vi "Monty-Hall.vi"() -> ()   [LabVIEW 2021]
uses:
  <vilib>/Platform/TimedLoop/XDataNode/timing_clust.ctl
  <vilib>/Platform/TimedLoop/XDataNode/nitl_modes.ctl
  <vilib>/Platform/TimedLoop/XDataNode/wakeup.ctl
  <vilib>/platform/TimedLoop/XDataNode/XDataNode.xnode
  <vilib>/Platform/TimedLoop/XDataNode/XDNodeRunTimeDep.lvlib
panel:
  out "Manual Wins":cluster{i32[], i32[]}[](graph)
  out "Manual Win":bool
  in  "Stay":bool
  in  "Switch":bool
  in  "?":bool
  in  "?":bool
  in  "?":bool
  in  "?":bool
  in  "?":bool
  in  "?":bool
  in  "?":bool
  in  "?":bool
  in  "?":bool
  in  "?":bool
  in  "Mode":i8(slide) min=0 max=2 step=1 scale=0.0..2.0
  out "Simulated Win":bool
  out "Simulated Odds":cluster{i32[], dbl[]}[](graph)
  in  "Door Count":dbl=3.0 min=3.0 max=10.0 step=1.0
  in  "Trial Count":dbl=1.0 min=1.0 step=1.0
  # "(note: set slider before starting VI)"
  # "In play mode, click a door, then either click switch or stay to remain with your original choice or swap to the other remaining door (Monty Hall Problem)"
  # "(note: VI automatically loops in play mode)"
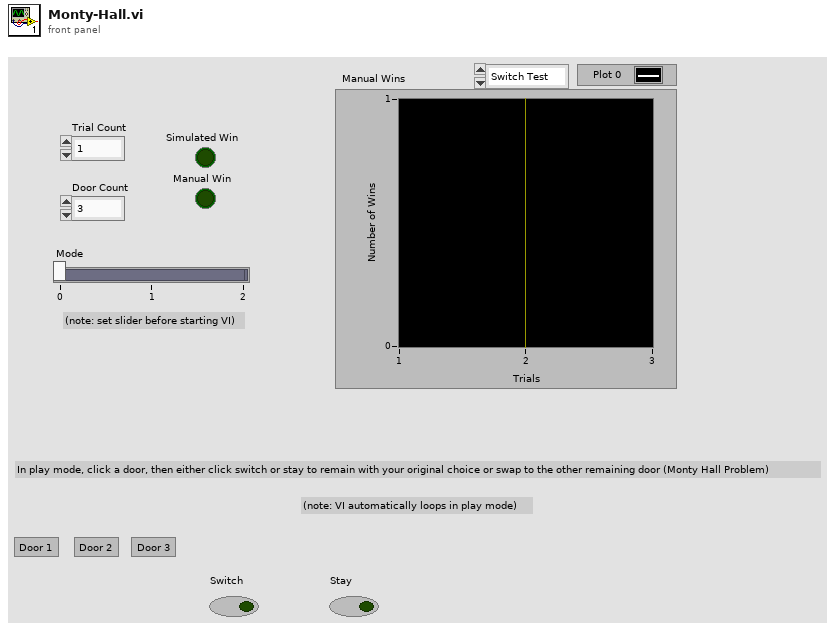
[diagram p1: front panel]
types:
  T1 = typedef "XDNodeRunTimeDep.lvlib/timing_clust.ctl" = cluster{"Expected End [f-1]":u64, "Actual End [f-1]":u64, "Finished Late? [f-1]":bool, "Expected End [i-1]":u64, "Actual End [i-1]":u64, "Finished Late? [i-1]":bool, "Expected Start [i]":u64, "Actual Start [i]":u64, "Expected Start [f]":u64, "Actual Start [f]":u64, "Source Name":string, "Structure Name":string, "Period":i64, "Deadline":i64, "Offset":i64, "Start":i64, "Priority":i32, "Timeout":i32, "Mode":T2, "Wakeup Reason":T3, "Error":errorcluster, "Source Type":string, "Secondary Source Type":string, "Global End Time":u64, "Global Start Time":u64, "Frame Duration":u64, "Iteration Duration":u64, "Assigned CPU":i32, "I/O Scan Engine Mode":u32}
  T2 = typedef "XDNodeRunTimeDep.lvlib/nitl_modes.ctl" = enum32{"No Change", "Process missed periods, maintain original phase", "Discard missed periods, maintain original phase", "Process missed periods, ignore original phase", "Discard missed periods, ignore original phase"}
  T3 = typedef "XDNodeRunTimeDep.lvlib/wakeup.ctl" = enum32{"Normal", "Aborted", "Asynchronous wakeup", "Timing source error", "Timed loop error", "Timeout"}
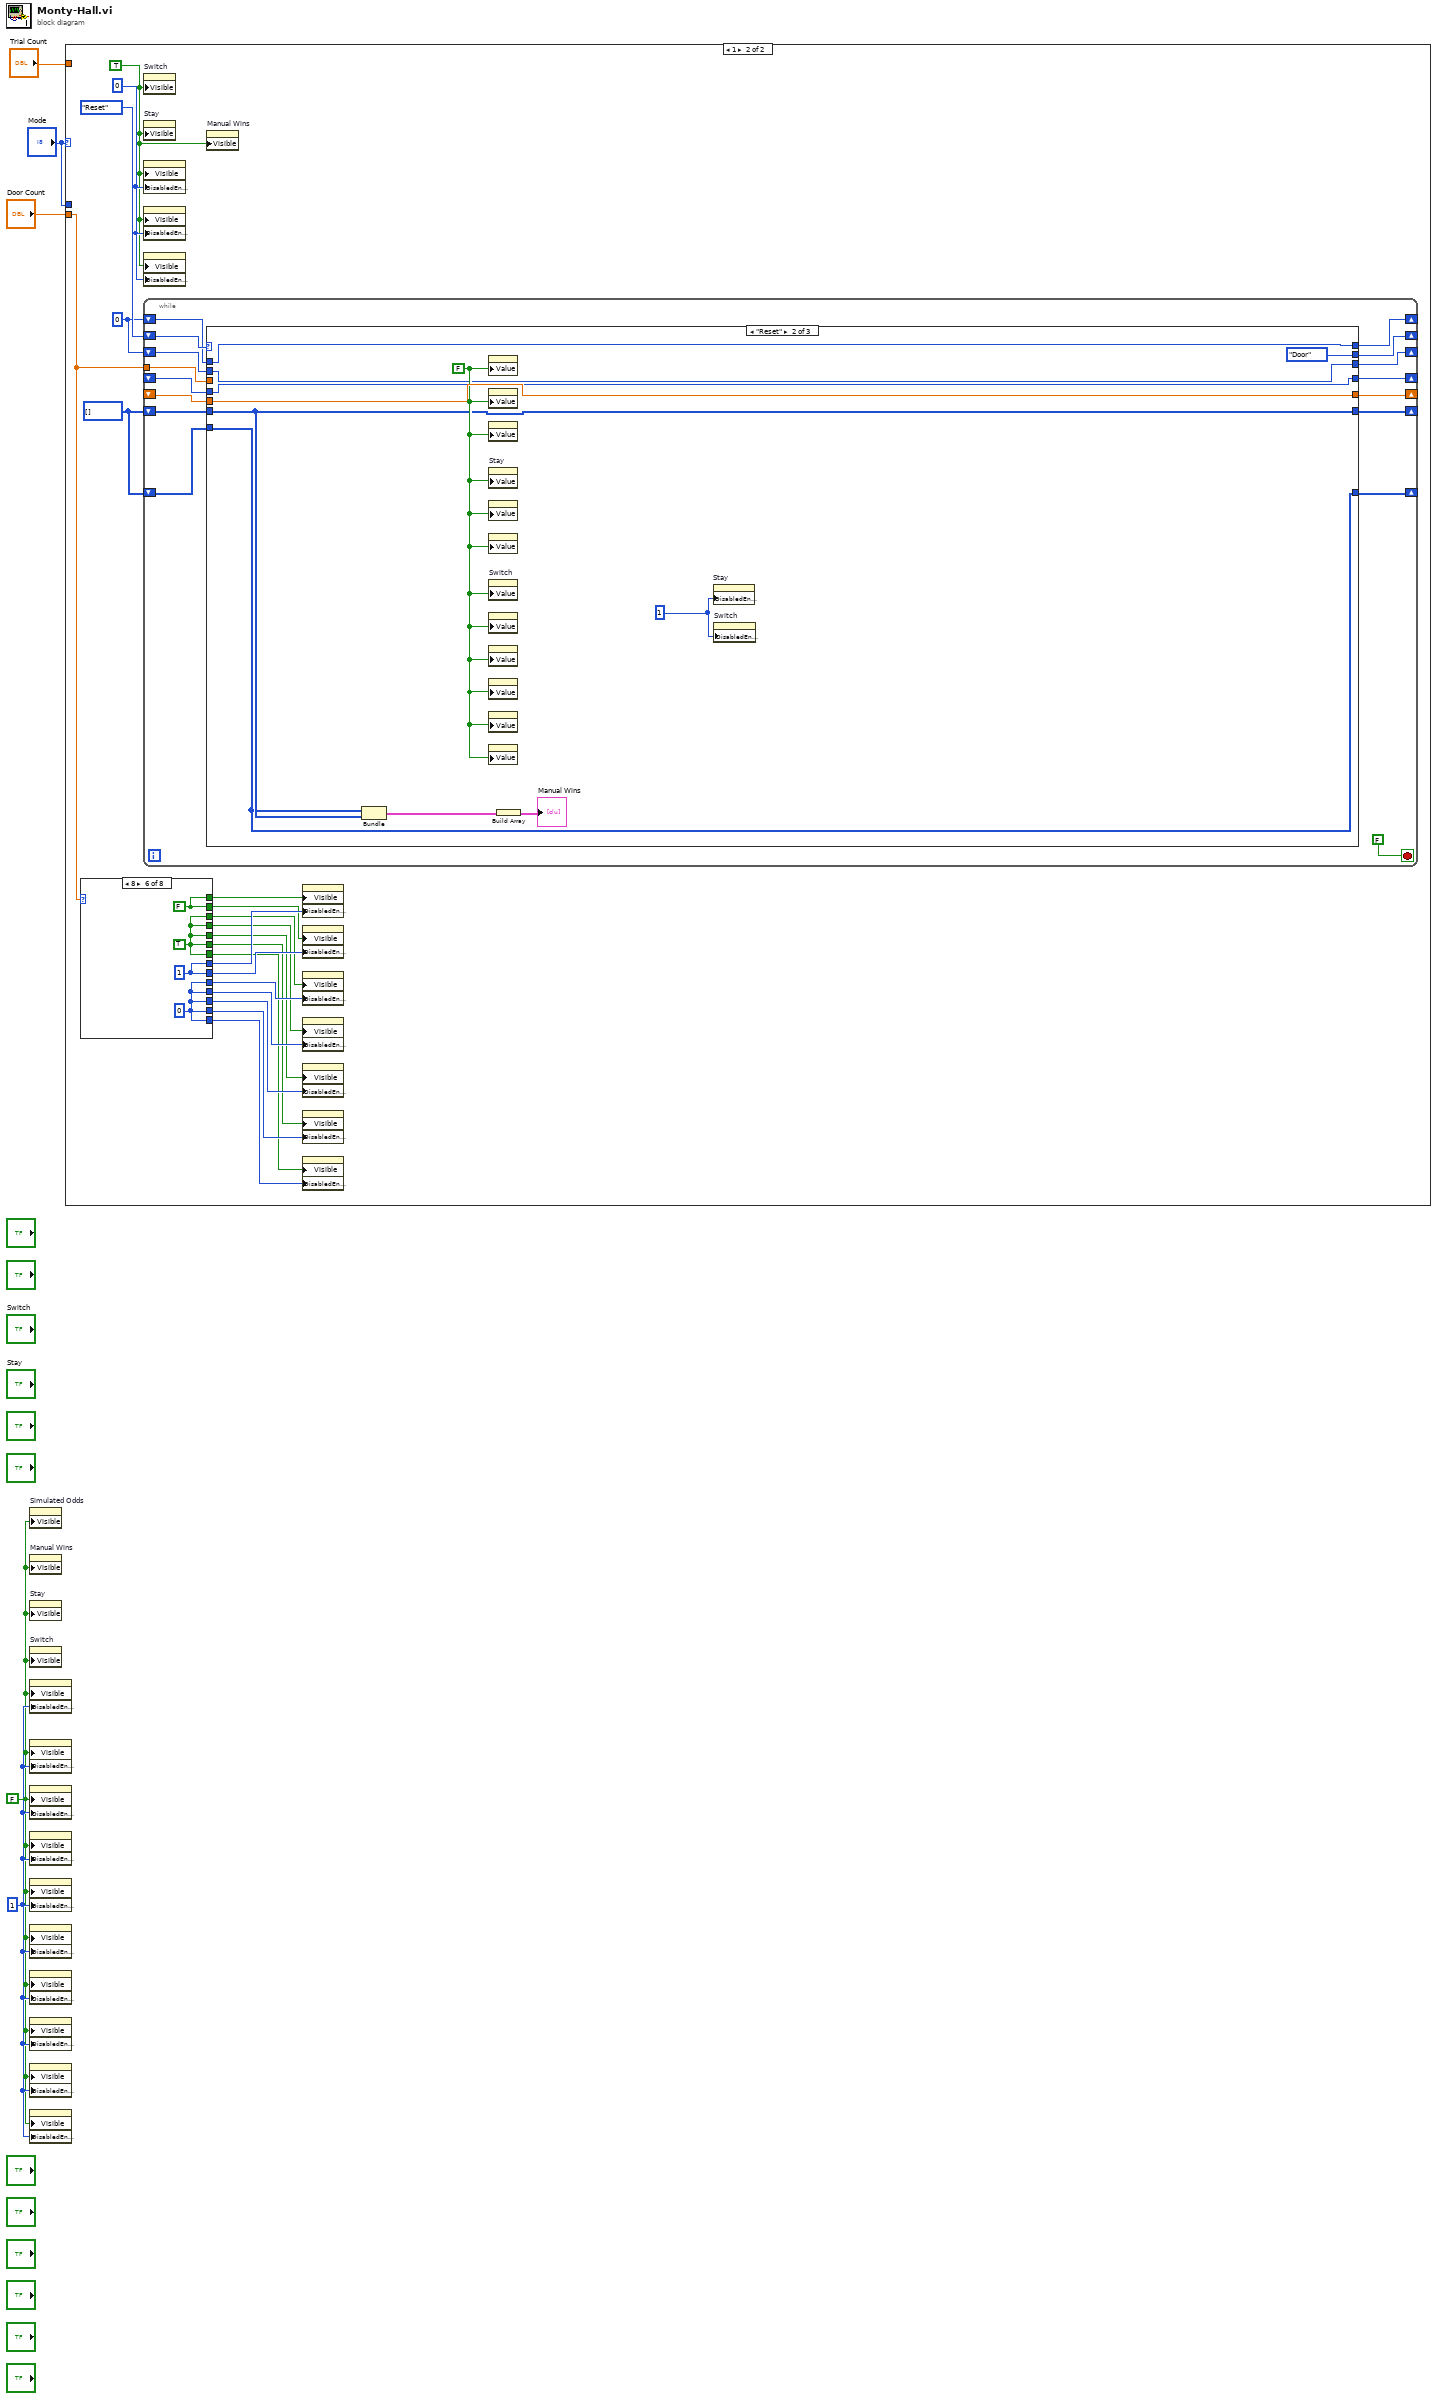
[diagram p0: block diagram]
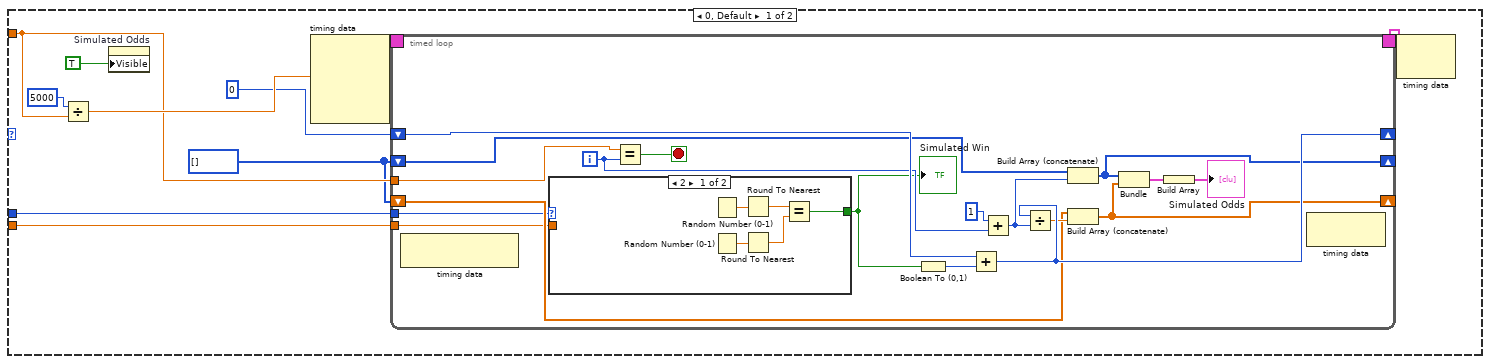
[diagram p2: hidden frame]
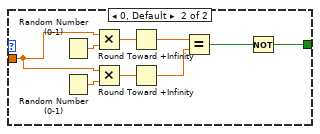
[diagram p3: hidden frame]
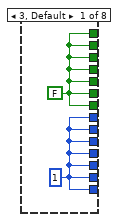
[diagram p4: hidden frame]
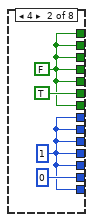
[diagram p5: hidden frame]
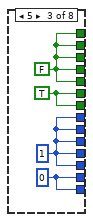
[diagram p6: hidden frame]
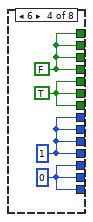
[diagram p7: hidden frame]
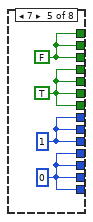
[diagram p8: hidden frame]
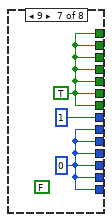
[diagram p9: hidden frame]
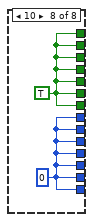
[diagram p10: hidden frame]
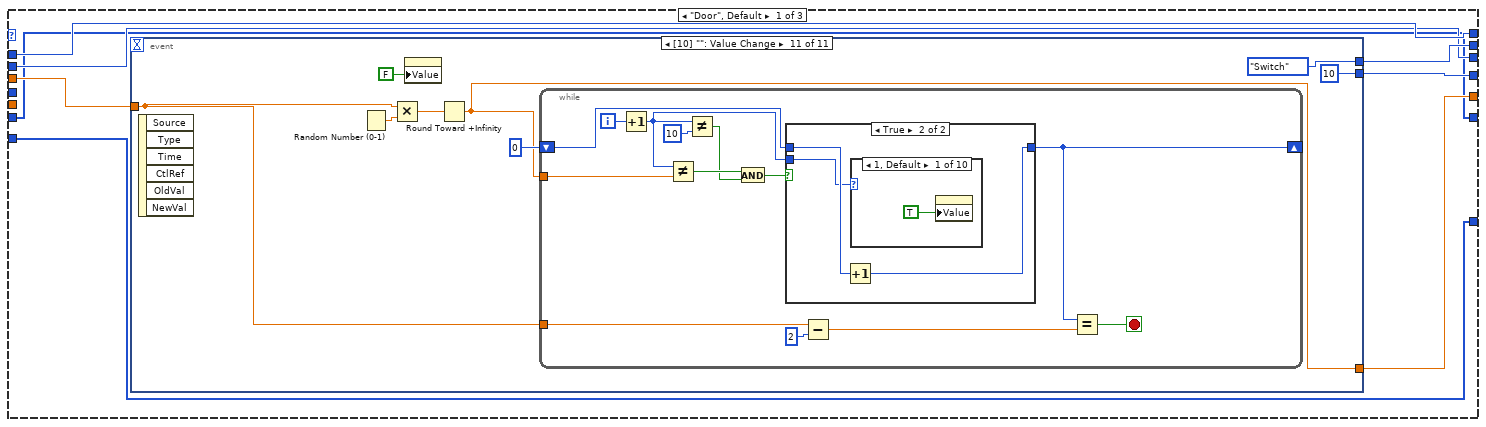
[diagram p11: hidden frame]
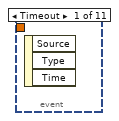
[diagram p12: hidden frame]
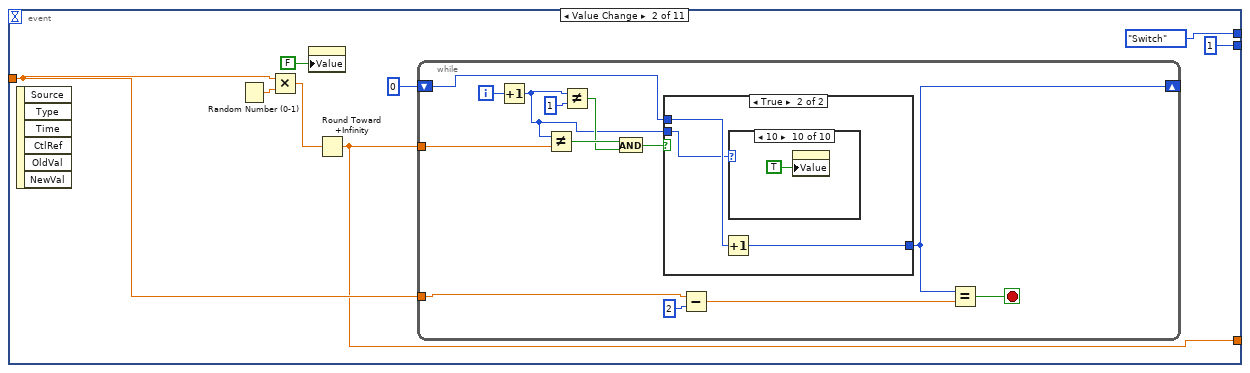
[diagram p13: hidden frame]
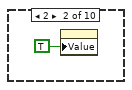
[diagram p16: hidden frame]
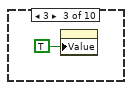
[diagram p17: hidden frame]
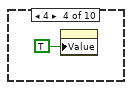
[diagram p18: hidden frame]
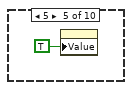
[diagram p19: hidden frame]
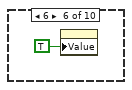
[diagram p20: hidden frame]
diagram:
  w3 = 1
  w1 = FALSE
  n1 = property on="Simulated Odds" class="XYGraph (strict)"("Visible"=w1) -> ()  [unwired: 2 in, 2 out]
  n2 = property on="Manual Wins" class="XYGraph (strict)"("Visible"=w1) -> ()  [unwired: 2 in, 2 out]
  n3 = property on="Stay" class="Bool (strict)"("Visible"=w1) -> ()  [unwired: 2 in, 2 out]
  n4 = property on="Switch" class="Bool (strict)"("Visible"=w1) -> ()  [unwired: 2 in, 2 out]
  n5 = property class="Bool (strict)"("Visible"=w1, "DisabledEnum"=w3) -> ()  [unwired: 2 in, 2 out]
  n6 = property class="Bool (strict)"("Visible"=w1, "DisabledEnum"=w3) -> ()  [unwired: 2 in, 2 out]
  n7 = property class="Bool (strict)"("Visible"=w1, "DisabledEnum"=w3) -> ()  [unwired: 2 in, 2 out]
  n8 = property class="Bool (strict)"("Visible"=w1, "DisabledEnum"=w3) -> ()  [unwired: 2 in, 2 out]
  n9 = property class="Bool (strict)"("Visible"=w1, "DisabledEnum"=w3) -> ()  [unwired: 2 in, 2 out]
  n10 = property class="Bool (strict)"("Visible"=w1, "DisabledEnum"=w3) -> ()  [unwired: 2 in, 2 out]
  n11 = property class="Bool (strict)"("Visible"=w1, "DisabledEnum"=w3) -> ()  [unwired: 2 in, 2 out]
  n12 = property class="Bool (strict)"("Visible"=w1, "DisabledEnum"=w3) -> ()  [unwired: 2 in, 2 out]
  n13 = property class="Bool (strict)"("Visible"=w1, "DisabledEnum"=w3) -> ()  [unwired: 2 in, 2 out]
  n14 = property class="Bool (strict)"("Visible"=w1, "DisabledEnum"=w3) -> ()  [unwired: 2 in, 2 out]
  n15 = case shown="1" "Mode" {
    tunnel: "Trial Count" -> [w11 _]
    tunnel: "Door Count" -> [w10 w72]
    tunnel: "Mode" -> [w7 _]
    frame 0, Default {
      w8 = i32[] []
      n16 = Divide(x=5000, y=w11) -> (x/y=w12:dbl)
      n17 = property on="Simulated Odds" class="XYGraph (strict)"("Visible"=TRUE) -> ()  [unwired: 2 in, 2 out]
      n18 = node-c288(w12) -> (w14:T1)  [unwired: 3 in]
      n19 = timed-loop {
        timing: w14 -> [_]
        timing-out: [_] -> w13
        shift-right: [w23] -> _
        shift-left: w8 -> [w22]
        tunnel: w11 -> [w33]
        tunnel: w10 -> [w18]
        shift-right: [w29] -> _
        shift-left: 0 -> [w30]
        shift-right: [w20] -> _
        shift-left: w8 -> [w19]
        tunnel: w7 -> [w16]
        i -> [w27]
        stop <- w32 stop-if-true
        n20 = node-c288() -> ()  [unwired: 1 in, 1 out]
        n21 = case shown="2" w16 {
          tunnel: w18 -> [_ w43]
          tunnel: [w34 w39] -> w17
          frame 2 {
            n22 = Random Number (0-1)() -> (number: 0 to 1=w38:dbl)
            n23 = Random Number (0-1)() -> (number: 0 to 1=w37:dbl)
            n24 = Round To Nearest(number=w38) -> (nearest integer value=w36:dbl)
            n25 = Round To Nearest(number=w37) -> (nearest integer value=w35:dbl)
            n26 = Equal?(x=w36, y=w35) -> (x = y?=w34:bool)
          }
          frame 0, Default {
            n27 = Random Number (0-1)() -> (number: 0 to 1=w47:dbl)
            n28 = Random Number (0-1)() -> (number: 0 to 1=w45:dbl)
            n29 = Multiply(x=w43, y=w47) -> (x*y=w46:dbl)
            n30 = Multiply(x=w43, y=w45) -> (x*y=w44:dbl)
            n31 = Round Toward +Infinity(x=w46) -> (ceil(x): smallest int >= x=w42:dbl)
            n32 = Round Toward +Infinity(x=w44) -> (ceil(x): smallest int >= x=w41:dbl)
            n33 = Equal?(x=w42, y=w41) -> (x = y?=w40:bool)
            n34 = Not(x=w40) -> (.not. x?=w39:bool)
          }
        }
        "Simulated Win" <- w17
        n35 = Equal?(x=w33, y=w27) -> (x = y?=w32:bool)
        n36 = Boolean To (0,1)(Boolean=w17) -> (0, 1=w31:i16)
        n37 = Add(x=w30, y=w31) -> (x+y=w29:i32)
        n38 = Add(x=1, y=w27) -> (x+y=w21:i32)
        n39 = Divide(x=w29, y=w21) -> (x/y=w24:dbl)
        n40 = Build Array (concatenate)(w19, w21) -> (w20:i32[])
        n41 = Build Array (concatenate)(w22, w24) -> (w23:dbl[])
        n42 = Bundle(w20, w23) -> (w26:cluster{i32[], dbl[]})  [unwired: 1 in]
        n43 = Build Array(w26) -> (→"Simulated Odds":cluster{i32[], dbl[]}[])
        n44 = node-c288() -> ()  [unwired: 1 in, 1 out]
      }
      n45 = node-c288(w13) -> ()  [unwired: 1 out]
    }
    frame 1 {
      w55 = i32[] []
      w56 = 0
      w54 = TRUE
      w73 = 0
      n46 = case shown="8" w72 {
        tunnel: [w75 0 w82 w87 w88 w92 w98 w99] -> w71
        tunnel: [w75 w77 w82 w87 w88 w92 w98 w99] -> w70
        tunnel: [w75 w77 w81 w87 w88 w92 w98 w99] -> w69
        tunnel: [w75 w77 w81 w85 w88 w92 w98 w99] -> w68
        tunnel: [w75 w77 w81 w85 w89 w92 w98 w99] -> w67
        tunnel: [w75 w77 w81 w85 w89 w94 w98 w99] -> w66
        tunnel: [w75 w77 w81 w85 w89 w94 1 w99] -> w65
        tunnel: [w74 TRUE w83 w86 w91 w95 w96 w100] -> w64
        tunnel: [w74 w76 w83 w86 w91 w95 w96 w100] -> w63
        tunnel: [w74 w76 w80 w86 w91 w95 w96 w100] -> w62
        tunnel: [w74 w76 w80 w84 w91 w95 w96 w100] -> w61
        tunnel: [w74 w76 w80 w84 w90 w95 w96 w100] -> w60
        tunnel: [w74 w76 w80 w84 w90 w93 w96 w100] -> w59
        tunnel: [w74 w76 w80 w84 w90 w93 w96 w100] -> w58
        frame 3, Default {
          w74 = FALSE
          w75 = 1
        }
        frame 4 {
          w76 = FALSE
          w77 = 1
        }
        frame 5 {
          w80 = FALSE
          w81 = 1
          w83 = TRUE
          w82 = 0
        }
        frame 6 {
          w84 = FALSE
          w85 = 1
          w86 = TRUE
          w87 = 0
        }
        frame 7 {
          w90 = FALSE
          w89 = 1
          w91 = TRUE
          w88 = 0
        }
        frame 8 {
          w93 = FALSE
          w94 = 1
          w95 = TRUE
          w92 = 0
        }
        frame 9 {
          (unwired) FALSE
          w96 = TRUE
          w98 = 0
        }
        frame 10 {
          w100 = TRUE
          w99 = 0
        }
      }
      n47 = property on="Switch" class="Bool (strict)"("Visible"=w54) -> ()  [unwired: 2 in, 2 out]
      n48 = property on="Stay" class="Bool (strict)"("Visible"=w54) -> ()  [unwired: 2 in, 2 out]
      n49 = property class="Bool (strict)"("Visible"=w54, "DisabledEnum"=w73) -> ()  [unwired: 2 in, 2 out]
      n50 = property class="Bool (strict)"("Visible"=w54, "DisabledEnum"=w73) -> ()  [unwired: 2 in, 2 out]
      n51 = property class="Bool (strict)"("Visible"=w54, "DisabledEnum"=w73) -> ()  [unwired: 2 in, 2 out]
      n52 = while {
        tunnel: w72 -> [w115]
        shift-right: [w113] -> _
        shift-left: enum16{"Door", "Reset", "Switch"}."Reset" -> [w114]
        shift-right: [w112] -> _
        shift-left: _ -> [w111]
        shift-right: [w110] -> _
        shift-left: _ -> [w109]
        shift-right: [w105] -> _
        shift-left: w56 -> [w106]
        shift-right: [w107] -> _
        shift-left: w56 -> [w108]
        shift-right: [w101] -> _
        shift-left: w55 -> [w104]
        shift-right: [w102] -> _
        shift-left: w55 -> [w103]
        stop <- FALSE stop-if-true
        n53 = case shown="\"Reset\"" w114 {
          tunnel: w115 -> [w124 _ _]
          tunnel: [w123 enum16{"Door", "Reset", "Switch"}."Door" enum16{"Door", "Reset", "Switch"}."Reset"] -> w113
          tunnel: [w122 w483 w497] -> w112
          tunnel: w111 -> [_ w483 w499]
          tunnel: [w121 w482 w497] -> w110
          tunnel: w109 -> [_ w482 w498]
          tunnel: w108 -> [w119 w478 w494]
          tunnel: [w119 w478 w489] -> w107
          tunnel: w106 -> [w120 w479 w492]
          tunnel: [w120 w479 w490] -> w105
          tunnel: w104 -> [w118 w475 w491]
          tunnel: w103 -> [w117 w476 w488]
          tunnel: [w117 w476 w487] -> w102
          tunnel: [w118 w475 w486] -> w101
          frame "Door", Default {
            n54 = event shown="[10] \"\": Value Change" {
              selector: _ -> [_ _ _ _ _ _ _ _ _ _ _]
              dyn-events: _ -> [_ _ _ _ _ _ _ _ _ _ _]
              timeout: _ -> [_ _ _ _ _ _ _ _ _ _ _]
              tunnel: w124 -> [_ w128 w159 w197 w232 w266 w301 w334 w371 w406 w441]
              tunnel: [_ enum16{"Door", "Reset", "Switch"}."Switch" enum16{"Door", "Reset", "Switch"}."Switch" enum16{"Door", "Reset", "Switch"}."Switch" enum16{"Door", "Reset", "Switch"}."Switch" enum16{"Door", "Reset", "Switch"}."Switch" enum16{"Door", "Reset", "Switch"}."Switch" enum16{"Door", "Reset", "Switch"}."Switch" enum16{"Door", "Reset", "Switch"}."Switch" enum16{"Door", "Reset", "Switch"}."Switch" enum16{"Door", "Reset", "Switch"}."Switch"] -> w123
              tunnel: [_ w127 w162 w196 w231 w267 w302 w337 w372 w407 w442] -> w122
              tunnel: [_ 1 2 3 4 5 6 7 8 9 10] -> w121
              event Timeout {
                n55 = event-data() -> ()  [unwired: 1 in, 3 out]
              }
              event Value Change {
                n56 = event-data() -> ()  [unwired: 1 in, 6 out]
                n57 = Random Number (0-1)() -> (number: 0 to 1=w131:dbl)
                n58 = Multiply(x=w128, y=w131) -> (x*y=w132:dbl)
                n59 = property class="Bool (strict)"("Value"=FALSE) -> ()  [unwired: 2 in, 2 out]
                n60 = Round Toward +Infinity(x=w132) -> (ceil(x): smallest int >= x=w127:dbl)
                n61 = while {
                  tunnel: w128 -> [w137]
                  tunnel: w127 -> [w145]
                  shift-right: [w139] -> _
                  shift-left: 0 -> [w140]
                  i -> [w134]
                  stop <- w135 stop-if-true
                  n62 = Increment(x=w134) -> (x+1=w133:i32)
                  n63 = Not Equal?(x=w133, y=w145) -> (x != y?=w144:bool)
                  n64 = Not Equal?(x=w133, y=1) -> (x != y?=w142:bool)
                  n65 = And(x=w144, y=w142) -> (x .and. y?=w141:bool)
                  n66 = case shown="True" w141 {
                    tunnel: w140 -> [w146 w149]
                    tunnel: [w146 w148] -> w139
                    tunnel: w133 -> [_ w147]
                    frame False {
                    }
                    frame True {
                      n67 = Increment(x=w149) -> (x+1=w148:i32)
                      n68 = case shown="10" w147 {
                        frame 1, Default {
                        }
                        frame 2 {
                          n69 = property class="Bool (strict)"("Value"=TRUE) -> ()  [unwired: 2 in, 2 out]
                        }
                        frame 3 {
                          n70 = property class="Bool (strict)"("Value"=TRUE) -> ()  [unwired: 2 in, 2 out]
                        }
                        frame 4 {
                          n71 = property class="Bool (strict)"("Value"=TRUE) -> ()  [unwired: 2 in, 2 out]
                        }
                        frame 5 {
                          n72 = property class="Bool (strict)"("Value"=TRUE) -> ()  [unwired: 2 in, 2 out]
                        }
                        frame 6 {
                          n73 = property class="Bool (strict)"("Value"=TRUE) -> ()  [unwired: 2 in, 2 out]
                        }
                        frame 7 {
                          n74 = property class="Bool (strict)"("Value"=TRUE) -> ()  [unwired: 2 in, 2 out]
                        }
                        frame 8 {
                          n75 = property class="Bool (strict)"("Value"=TRUE) -> ()  [unwired: 2 in, 2 out]
                        }
                        frame 9 {
                          n76 = property class="Bool (strict)"("Value"=TRUE) -> ()  [unwired: 2 in, 2 out]
                        }
                        frame 10 {
                          n77 = property class="Bool (strict)"("Value"=TRUE) -> ()  [unwired: 2 in, 2 out]
                        }
                      }
                    }
                  }
                  n78 = Subtract(x=w137, y=2) -> (x-y=w136:dbl)
                  n79 = Equal?(x=w139, y=w136) -> (x = y?=w135:bool)
                }
              }
              event Value Change {
                n80 = event-data() -> ()  [unwired: 1 in, 6 out]
                n81 = Random Number (0-1)() -> (number: 0 to 1=w165:dbl)
                n82 = Multiply(x=w159, y=w165) -> (x*y=w166:dbl)
                n83 = property class="Bool (strict)"("Value"=FALSE) -> ()  [unwired: 2 in, 2 out]
                n84 = Round Toward +Infinity(x=w166) -> (ceil(x): smallest int >= x=w162:dbl)
                n85 = while {
                  tunnel: w159 -> [w171]
                  tunnel: w162 -> [w179]
                  shift-right: [w173] -> _
                  shift-left: 0 -> [w174]
                  i -> [w168]
                  stop <- w169 stop-if-true
                  n86 = Increment(x=w168) -> (x+1=w167:i32)
                  n87 = Not Equal?(x=w167, y=w179) -> (x != y?=w178:bool)
                  n88 = Not Equal?(x=w167, y=2) -> (x != y?=w176:bool)
                  n89 = And(x=w178, y=w176) -> (x .and. y?=w175:bool)
                  n90 = case shown="True" w175 {
                    tunnel: w174 -> [w180 w183]
                    tunnel: [w180 w182] -> w173
                    tunnel: w167 -> [_ w181]
                    frame False {
                    }
                    frame True {
                      n91 = Increment(x=w183) -> (x+1=w182:i32)
                      n92 = case shown="10" w181 {
                        frame 1, Default {
                          n93 = property class="Bool (strict)"("Value"=TRUE) -> ()  [unwired: 2 in, 2 out]
                        }
                        frame 2 {
                          n94 = property class="Bool (strict)"("Value"=TRUE) -> ()  [unwired: 2 in, 2 out]
                        }
                        frame 3 {
                          n95 = property class="Bool (strict)"("Value"=TRUE) -> ()  [unwired: 2 in, 2 out]
                        }
                        frame 4 {
                          n96 = property class="Bool (strict)"("Value"=TRUE) -> ()  [unwired: 2 in, 2 out]
                        }
                        frame 5 {
                          n97 = property class="Bool (strict)"("Value"=TRUE) -> ()  [unwired: 2 in, 2 out]
                        }
                        frame 6 {
                          n98 = property class="Bool (strict)"("Value"=TRUE) -> ()  [unwired: 2 in, 2 out]
                        }
                        frame 7 {
                          n99 = property class="Bool (strict)"("Value"=TRUE) -> ()  [unwired: 2 in, 2 out]
                        }
                        frame 8 {
                          n100 = property class="Bool (strict)"("Value"=TRUE) -> ()  [unwired: 2 in, 2 out]
                        }
                        frame 9 {
                          n101 = property class="Bool (strict)"("Value"=TRUE) -> ()  [unwired: 2 in, 2 out]
                        }
                        frame 10 {
                          n102 = property class="Bool (strict)"("Value"=TRUE) -> ()  [unwired: 2 in, 2 out]
                        }
                      }
                    }
                  }
                  n103 = Subtract(x=w171, y=2) -> (x-y=w170:dbl)
                  n104 = Equal?(x=w173, y=w170) -> (x = y?=w169:bool)
                }
              }
              event Value Change {
                n105 = event-data() -> ()  [unwired: 1 in, 6 out]
                n106 = Random Number (0-1)() -> (number: 0 to 1=w200:dbl)
                n107 = Multiply(x=w197, y=w200) -> (x*y=w201:dbl)
                n108 = property class="Bool (strict)"("Value"=FALSE) -> ()  [unwired: 2 in, 2 out]
                n109 = Round Toward +Infinity(x=w201) -> (ceil(x): smallest int >= x=w196:dbl)
                n110 = while {
                  tunnel: w197 -> [w206]
                  tunnel: w196 -> [w214]
                  shift-right: [w208] -> _
                  shift-left: 0 -> [w209]
                  i -> [w203]
                  stop <- w204 stop-if-true
                  n111 = Increment(x=w203) -> (x+1=w202:i32)
                  n112 = Not Equal?(x=w202, y=w214) -> (x != y?=w213:bool)
                  n113 = Not Equal?(x=w202, y=3) -> (x != y?=w211:bool)
                  n114 = And(x=w213, y=w211) -> (x .and. y?=w210:bool)
                  n115 = case shown="True" w210 {
                    tunnel: w209 -> [w215 w218]
                    tunnel: [w215 w217] -> w208
                    tunnel: w202 -> [_ w216]
                    frame False {
                    }
                    frame True {
                      n116 = Increment(x=w218) -> (x+1=w217:i32)
                      n117 = case shown="1, Default" w216 {
                        frame 1, Default {
                          n118 = property class="Bool (strict)"("Value"=TRUE) -> ()  [unwired: 2 in, 2 out]
                        }
                        frame 2 {
                          n119 = property class="Bool (strict)"("Value"=TRUE) -> ()  [unwired: 2 in, 2 out]
                        }
                        frame 3 {
                          n120 = property class="Bool (strict)"("Value"=TRUE) -> ()  [unwired: 2 in, 2 out]
                        }
                        frame 4 {
                          n121 = property class="Bool (strict)"("Value"=TRUE) -> ()  [unwired: 2 in, 2 out]
                        }
                        frame 5 {
                          n122 = property class="Bool (strict)"("Value"=TRUE) -> ()  [unwired: 2 in, 2 out]
                        }
                        frame 6 {
                          n123 = property class="Bool (strict)"("Value"=TRUE) -> ()  [unwired: 2 in, 2 out]
                        }
                        frame 7 {
                          n124 = property class="Bool (strict)"("Value"=TRUE) -> ()  [unwired: 2 in, 2 out]
                        }
                        frame 8 {
                          n125 = property class="Bool (strict)"("Value"=TRUE) -> ()  [unwired: 2 in, 2 out]
                        }
                        frame 9 {
                          n126 = property class="Bool (strict)"("Value"=TRUE) -> ()  [unwired: 2 in, 2 out]
                        }
                        frame 10 {
                          n127 = property class="Bool (strict)"("Value"=TRUE) -> ()  [unwired: 2 in, 2 out]
                        }
                      }
                    }
                  }
                  n128 = Subtract(x=w206, y=2) -> (x-y=w205:dbl)
                  n129 = Equal?(x=w208, y=w205) -> (x = y?=w204:bool)
                }
              }
              event Value Change {
                n130 = event-data() -> ()  [unwired: 1 in, 6 out]
                n131 = Random Number (0-1)() -> (number: 0 to 1=w236:dbl)
                n132 = Multiply(x=w232, y=w236) -> (x*y=w235:dbl)
                n133 = property class="Bool (strict)"("Value"=FALSE) -> ()  [unwired: 2 in, 2 out]
                n134 = Round Toward +Infinity(x=w235) -> (ceil(x): smallest int >= x=w231:dbl)
                n135 = while {
                  tunnel: w232 -> [w241]
                  tunnel: w231 -> [w249]
                  shift-right: [w243] -> _
                  shift-left: 0 -> [w244]
                  i -> [w238]
                  stop <- w239 stop-if-true
                  n136 = Increment(x=w238) -> (x+1=w237:i32)
                  n137 = Not Equal?(x=w237, y=w249) -> (x != y?=w248:bool)
                  n138 = Not Equal?(x=w237, y=4) -> (x != y?=w246:bool)
                  n139 = And(x=w248, y=w246) -> (x .and. y?=w245:bool)
                  n140 = case shown="True" w245 {
                    tunnel: w244 -> [w250 w253]
                    tunnel: [w250 w252] -> w243
                    tunnel: w237 -> [_ w251]
                    frame False {
                    }
                    frame True {
                      n141 = Increment(x=w253) -> (x+1=w252:i32)
                      n142 = case shown="1, Default" w251 {
                        frame 1, Default {
                          n143 = property class="Bool (strict)"("Value"=TRUE) -> ()  [unwired: 2 in, 2 out]
                        }
                        frame 2 {
                          n144 = property class="Bool (strict)"("Value"=TRUE) -> ()  [unwired: 2 in, 2 out]
                        }
                        frame 3 {
                          n145 = property class="Bool (strict)"("Value"=TRUE) -> ()  [unwired: 2 in, 2 out]
                        }
                        frame 4 {
                          n146 = property class="Bool (strict)"("Value"=TRUE) -> ()  [unwired: 2 in, 2 out]
                        }
                        frame 5 {
                          n147 = property class="Bool (strict)"("Value"=TRUE) -> ()  [unwired: 2 in, 2 out]
                        }
                        frame 6 {
                          n148 = property class="Bool (strict)"("Value"=TRUE) -> ()  [unwired: 2 in, 2 out]
                        }
                        frame 7 {
                          n149 = property class="Bool (strict)"("Value"=TRUE) -> ()  [unwired: 2 in, 2 out]
                        }
                        frame 8 {
                          n150 = property class="Bool (strict)"("Value"=TRUE) -> ()  [unwired: 2 in, 2 out]
                        }
                        frame 9 {
                          n151 = property class="Bool (strict)"("Value"=TRUE) -> ()  [unwired: 2 in, 2 out]
                        }
                        frame 10 {
                          n152 = property class="Bool (strict)"("Value"=TRUE) -> ()  [unwired: 2 in, 2 out]
                        }
                      }
                    }
                  }
                  n153 = Subtract(x=w241, y=2) -> (x-y=w240:dbl)
                  n154 = Equal?(x=w243, y=w240) -> (x = y?=w239:bool)
                }
              }
              event Value Change {
                n155 = event-data() -> ()  [unwired: 1 in, 6 out]
                n156 = Random Number (0-1)() -> (number: 0 to 1=w270:dbl)
                n157 = Multiply(x=w266, y=w270) -> (x*y=w271:dbl)
                n158 = property class="Bool (strict)"("Value"=FALSE) -> ()  [unwired: 2 in, 2 out]
                n159 = Round Toward +Infinity(x=w271) -> (ceil(x): smallest int >= x=w267:dbl)
                n160 = while {
                  tunnel: w267 -> [w284]
                  shift-right: [w278] -> _
                  shift-left: 0 -> [w279]
                  tunnel: w266 -> [w272]
                  i -> [w274]
                  stop <- w275 stop-if-true
                  n161 = Increment(x=w274) -> (x+1=w273:i32)
                  n162 = Not Equal?(x=w273, y=w284) -> (x != y?=w283:bool)
                  n163 = Not Equal?(x=w273, y=5) -> (x != y?=w281:bool)
                  n164 = And(x=w283, y=w281) -> (x .and. y?=w280:bool)
                  n165 = case shown="True" w280 {
                    tunnel: w279 -> [w285 w288]
                    tunnel: [w285 w287] -> w278
                    tunnel: w273 -> [_ w286]
                    frame False {
                    }
                    frame True {
                      n166 = case shown="1, Default" w286 {
                        frame 1, Default {
                          n167 = property class="Bool (strict)"("Value"=TRUE) -> ()  [unwired: 2 in, 2 out]
                        }
                        frame 2 {
                          n168 = property class="Bool (strict)"("Value"=TRUE) -> ()  [unwired: 2 in, 2 out]
                        }
                        frame 3 {
                          n169 = property class="Bool (strict)"("Value"=TRUE) -> ()  [unwired: 2 in, 2 out]
                        }
                        frame 4 {
                          n170 = property class="Bool (strict)"("Value"=TRUE) -> ()  [unwired: 2 in, 2 out]
                        }
                        frame 5 {
                          n171 = property class="Bool (strict)"("Value"=TRUE) -> ()  [unwired: 2 in, 2 out]
                        }
                        frame 6 {
                          n172 = property class="Bool (strict)"("Value"=TRUE) -> ()  [unwired: 2 in, 2 out]
                        }
                        frame 7 {
                          n173 = property class="Bool (strict)"("Value"=TRUE) -> ()  [unwired: 2 in, 2 out]
                        }
                        frame 8 {
                          n174 = property class="Bool (strict)"("Value"=TRUE) -> ()  [unwired: 2 in, 2 out]
                        }
                        frame 9 {
                          n175 = property class="Bool (strict)"("Value"=TRUE) -> ()  [unwired: 2 in, 2 out]
                        }
                        frame 10 {
                          n176 = property class="Bool (strict)"("Value"=TRUE) -> ()  [unwired: 2 in, 2 out]
                        }
                      }
                      n177 = Increment(x=w288) -> (x+1=w287:i32)
                    }
                  }
                  n178 = Subtract(x=w272, y=2) -> (x-y=w276:dbl)
                  n179 = Equal?(x=w278, y=w276) -> (x = y?=w275:bool)
                }
              }
              event Value Change {
                n180 = event-data() -> ()  [unwired: 1 in, 6 out]
                n181 = Random Number (0-1)() -> (number: 0 to 1=w306:dbl)
                n182 = Multiply(x=w301, y=w306) -> (x*y=w305:dbl)
                n183 = property class="Bool (strict)"("Value"=FALSE) -> ()  [unwired: 2 in, 2 out]
                n184 = Round Toward +Infinity(x=w305) -> (ceil(x): smallest int >= x=w302:dbl)
                n185 = while {
                  tunnel: w302 -> [w319]
                  shift-right: [w313] -> _
                  shift-left: 0 -> [w314]
                  tunnel: w301 -> [w307]
                  i -> [w309]
                  stop <- w310 stop-if-true
                  n186 = Increment(x=w309) -> (x+1=w308:i32)
                  n187 = Not Equal?(x=w308, y=w319) -> (x != y?=w318:bool)
                  n188 = Not Equal?(x=w308, y=6) -> (x != y?=w316:bool)
                  n189 = And(x=w318, y=w316) -> (x .and. y?=w315:bool)
                  n190 = case shown="True" w315 {
                    tunnel: w314 -> [w320 w323]
                    tunnel: [w320 w322] -> w313
                    tunnel: w308 -> [_ w321]
                    frame False {
                    }
                    frame True {
                      n191 = Increment(x=w323) -> (x+1=w322:i32)
                      n192 = case shown="1, Default" w321 {
                        frame 1, Default {
                          n193 = property class="Bool (strict)"("Value"=TRUE) -> ()  [unwired: 2 in, 2 out]
                        }
                        frame 2 {
                          n194 = property class="Bool (strict)"("Value"=TRUE) -> ()  [unwired: 2 in, 2 out]
                        }
                        frame 3 {
                          n195 = property class="Bool (strict)"("Value"=TRUE) -> ()  [unwired: 2 in, 2 out]
                        }
                        frame 4 {
                          n196 = property class="Bool (strict)"("Value"=TRUE) -> ()  [unwired: 2 in, 2 out]
                        }
                        frame 5 {
                          n197 = property class="Bool (strict)"("Value"=TRUE) -> ()  [unwired: 2 in, 2 out]
                        }
                        frame 6 {
                          n198 = property class="Bool (strict)"("Value"=TRUE) -> ()  [unwired: 2 in, 2 out]
                        }
                        frame 7 {
                          n199 = property class="Bool (strict)"("Value"=TRUE) -> ()  [unwired: 2 in, 2 out]
                        }
                        frame 8 {
                          n200 = property class="Bool (strict)"("Value"=TRUE) -> ()  [unwired: 2 in, 2 out]
                        }
                        frame 9 {
                          n201 = property class="Bool (strict)"("Value"=TRUE) -> ()  [unwired: 2 in, 2 out]
                        }
                        frame 10 {
                          n202 = property class="Bool (strict)"("Value"=TRUE) -> ()  [unwired: 2 in, 2 out]
                        }
                      }
                    }
                  }
                  n203 = Subtract(x=w307, y=2) -> (x-y=w311:dbl)
                  n204 = Equal?(x=w313, y=w311) -> (x = y?=w310:bool)
                }
              }
              event Value Change {
                n205 = event-data() -> ()  [unwired: 1 in, 6 out]
                n206 = Random Number (0-1)() -> (number: 0 to 1=w341:dbl)
                n207 = Multiply(x=w334, y=w341) -> (x*y=w340:dbl)
                n208 = property class="Bool (strict)"("Value"=FALSE) -> ()  [unwired: 2 in, 2 out]
                n209 = Round Toward +Infinity(x=w340) -> (ceil(x): smallest int >= x=w337:dbl)
                n210 = while {
                  tunnel: w337 -> [w354]
                  shift-right: [w348] -> _
                  shift-left: 0 -> [w349]
                  tunnel: w334 -> [w342]
                  i -> [w344]
                  stop <- w345 stop-if-true
                  n211 = Increment(x=w344) -> (x+1=w343:i32)
                  n212 = Not Equal?(x=w343, y=w354) -> (x != y?=w353:bool)
                  n213 = Not Equal?(x=w343, y=7) -> (x != y?=w351:bool)
                  n214 = And(x=w353, y=w351) -> (x .and. y?=w350:bool)
                  n215 = case shown="True" w350 {
                    tunnel: w349 -> [w355 w358]
                    tunnel: [w355 w357] -> w348
                    tunnel: w343 -> [_ w356]
                    frame False {
                    }
                    frame True {
                      n216 = Increment(x=w358) -> (x+1=w357:i32)
                      n217 = case shown="1, Default" w356 {
                        frame 1, Default {
                          n218 = property class="Bool (strict)"("Value"=TRUE) -> ()  [unwired: 2 in, 2 out]
                        }
                        frame 2 {
                          n219 = property class="Bool (strict)"("Value"=TRUE) -> ()  [unwired: 2 in, 2 out]
                        }
                        frame 3 {
                          n220 = property class="Bool (strict)"("Value"=TRUE) -> ()  [unwired: 2 in, 2 out]
                        }
                        frame 4 {
                          n221 = property class="Bool (strict)"("Value"=TRUE) -> ()  [unwired: 2 in, 2 out]
                        }
                        frame 5 {
                          n222 = property class="Bool (strict)"("Value"=TRUE) -> ()  [unwired: 2 in, 2 out]
                        }
                        frame 6 {
                          n223 = property class="Bool (strict)"("Value"=TRUE) -> ()  [unwired: 2 in, 2 out]
                        }
                        frame 7 {
                          n224 = property class="Bool (strict)"("Value"=TRUE) -> ()  [unwired: 2 in, 2 out]
                        }
                        frame 8 {
                          n225 = property class="Bool (strict)"("Value"=TRUE) -> ()  [unwired: 2 in, 2 out]
                        }
                        frame 9 {
                          n226 = property class="Bool (strict)"("Value"=TRUE) -> ()  [unwired: 2 in, 2 out]
                        }
                        frame 10 {
                          n227 = property class="Bool (strict)"("Value"=TRUE) -> ()  [unwired: 2 in, 2 out]
                        }
                      }
                    }
                  }
                  n228 = Subtract(x=w342, y=2) -> (x-y=w346:dbl)
                  n229 = Equal?(x=w348, y=w346) -> (x = y?=w345:bool)
                }
              }
              event Value Change {
                n230 = event-data() -> ()  [unwired: 1 in, 6 out]
                n231 = Random Number (0-1)() -> (number: 0 to 1=w376:dbl)
                n232 = Multiply(x=w371, y=w376) -> (x*y=w375:dbl)
                n233 = property class="Bool (strict)"("Value"=FALSE) -> ()  [unwired: 2 in, 2 out]
                n234 = Round Toward +Infinity(x=w375) -> (ceil(x): smallest int >= x=w372:dbl)
                n235 = while {
                  tunnel: w372 -> [w389]
                  shift-right: [w383] -> _
                  shift-left: 0 -> [w384]
                  tunnel: w371 -> [w377]
                  i -> [w379]
                  stop <- w380 stop-if-true
                  n236 = Increment(x=w379) -> (x+1=w378:i32)
                  n237 = Not Equal?(x=w378, y=w389) -> (x != y?=w388:bool)
                  n238 = Not Equal?(x=w378, y=8) -> (x != y?=w386:bool)
                  n239 = And(x=w388, y=w386) -> (x .and. y?=w385:bool)
                  n240 = case shown="True" w385 {
                    tunnel: w384 -> [w390 w393]
                    tunnel: [w390 w392] -> w383
                    tunnel: w378 -> [_ w391]
                    frame False {
                    }
                    frame True {
                      n241 = Increment(x=w393) -> (x+1=w392:i32)
                      n242 = case shown="1, Default" w391 {
                        frame 1, Default {
                          n243 = property class="Bool (strict)"("Value"=TRUE) -> ()  [unwired: 2 in, 2 out]
                        }
                        frame 2 {
                          n244 = property class="Bool (strict)"("Value"=TRUE) -> ()  [unwired: 2 in, 2 out]
                        }
                        frame 3 {
                          n245 = property class="Bool (strict)"("Value"=TRUE) -> ()  [unwired: 2 in, 2 out]
                        }
                        frame 4 {
                          n246 = property class="Bool (strict)"("Value"=TRUE) -> ()  [unwired: 2 in, 2 out]
                        }
                        frame 5 {
                          n247 = property class="Bool (strict)"("Value"=TRUE) -> ()  [unwired: 2 in, 2 out]
                        }
                        frame 6 {
                          n248 = property class="Bool (strict)"("Value"=TRUE) -> ()  [unwired: 2 in, 2 out]
                        }
                        frame 7 {
                          n249 = property class="Bool (strict)"("Value"=TRUE) -> ()  [unwired: 2 in, 2 out]
                        }
                        frame 8 {
                          n250 = property class="Bool (strict)"("Value"=TRUE) -> ()  [unwired: 2 in, 2 out]
                        }
                        frame 9 {
                          n251 = property class="Bool (strict)"("Value"=TRUE) -> ()  [unwired: 2 in, 2 out]
                        }
                        frame 10 {
                          n252 = property class="Bool (strict)"("Value"=TRUE) -> ()  [unwired: 2 in, 2 out]
                        }
                      }
                    }
                  }
                  n253 = Subtract(x=w377, y=2) -> (x-y=w381:dbl)
                  n254 = Equal?(x=w383, y=w381) -> (x = y?=w380:bool)
                }
              }
              event Value Change {
                n255 = event-data() -> ()  [unwired: 1 in, 6 out]
                n256 = Random Number (0-1)() -> (number: 0 to 1=w411:dbl)
                n257 = Multiply(x=w406, y=w411) -> (x*y=w410:dbl)
                n258 = property class="Bool (strict)"("Value"=FALSE) -> ()  [unwired: 2 in, 2 out]
                n259 = Round Toward +Infinity(x=w410) -> (ceil(x): smallest int >= x=w407:dbl)
                n260 = while {
                  tunnel: w407 -> [w424]
                  shift-right: [w418] -> _
                  shift-left: 0 -> [w419]
                  tunnel: w406 -> [w412]
                  i -> [w414]
                  stop <- w415 stop-if-true
                  n261 = Increment(x=w414) -> (x+1=w413:i32)
                  n262 = Not Equal?(x=w413, y=w424) -> (x != y?=w423:bool)
                  n263 = Not Equal?(x=w413, y=9) -> (x != y?=w421:bool)
                  n264 = And(x=w423, y=w421) -> (x .and. y?=w420:bool)
                  n265 = case shown="True" w420 {
                    tunnel: w419 -> [w425 w428]
                    tunnel: [w425 w427] -> w418
                    tunnel: w413 -> [_ w426]
                    frame False {
                    }
                    frame True {
                      n266 = Increment(x=w428) -> (x+1=w427:i32)
                      n267 = case shown="1, Default" w426 {
                        frame 1, Default {
                          n268 = property class="Bool (strict)"("Value"=TRUE) -> ()  [unwired: 2 in, 2 out]
                        }
                        frame 2 {
                          n269 = property class="Bool (strict)"("Value"=TRUE) -> ()  [unwired: 2 in, 2 out]
                        }
                        frame 3 {
                          n270 = property class="Bool (strict)"("Value"=TRUE) -> ()  [unwired: 2 in, 2 out]
                        }
                        frame 4 {
                          n271 = property class="Bool (strict)"("Value"=TRUE) -> ()  [unwired: 2 in, 2 out]
                        }
                        frame 5 {
                          n272 = property class="Bool (strict)"("Value"=TRUE) -> ()  [unwired: 2 in, 2 out]
                        }
                        frame 6 {
                          n273 = property class="Bool (strict)"("Value"=TRUE) -> ()  [unwired: 2 in, 2 out]
                        }
                        frame 7 {
                          n274 = property class="Bool (strict)"("Value"=TRUE) -> ()  [unwired: 2 in, 2 out]
                        }
                        frame 8 {
                          n275 = property class="Bool (strict)"("Value"=TRUE) -> ()  [unwired: 2 in, 2 out]
                        }
                        frame 9 {
                          n276 = property class="Bool (strict)"("Value"=TRUE) -> ()  [unwired: 2 in, 2 out]
                        }
                        frame 10 {
                          n277 = property class="Bool (strict)"("Value"=TRUE) -> ()  [unwired: 2 in, 2 out]
                        }
                      }
                    }
                  }
                  n278 = Subtract(x=w412, y=2) -> (x-y=w416:dbl)
                  n279 = Equal?(x=w418, y=w416) -> (x = y?=w415:bool)
                }
              }
              event Value Change {
                n280 = event-data() -> ()  [unwired: 1 in, 6 out]
                n281 = Random Number (0-1)() -> (number: 0 to 1=w446:dbl)
                n282 = Multiply(x=w441, y=w446) -> (x*y=w445:dbl)
                n283 = property class="Bool (strict)"("Value"=FALSE) -> ()  [unwired: 2 in, 2 out]
                n284 = Round Toward +Infinity(x=w445) -> (ceil(x): smallest int >= x=w442:dbl)
                n285 = while {
                  tunnel: w442 -> [w459]
                  shift-right: [w453] -> _
                  shift-left: 0 -> [w454]
                  tunnel: w441 -> [w447]
                  i -> [w449]
                  stop <- w450 stop-if-true
                  n286 = Increment(x=w449) -> (x+1=w448:i32)
                  n287 = Not Equal?(x=w448, y=w459) -> (x != y?=w458:bool)
                  n288 = Not Equal?(x=w448, y=10) -> (x != y?=w456:bool)
                  n289 = And(x=w458, y=w456) -> (x .and. y?=w455:bool)
                  n290 = case shown="True" w455 {
                    tunnel: w454 -> [w460 w463]
                    tunnel: [w460 w462] -> w453
                    tunnel: w448 -> [_ w461]
                    frame False {
                    }
                    frame True {
                      n291 = Increment(x=w463) -> (x+1=w462:i32)
                      n292 = case shown="1, Default" w461 {
                        frame 1, Default {
                          n293 = property class="Bool (strict)"("Value"=TRUE) -> ()  [unwired: 2 in, 2 out]
                        }
                        frame 2 {
                          n294 = property class="Bool (strict)"("Value"=TRUE) -> ()  [unwired: 2 in, 2 out]
                        }
                        frame 3 {
                          n295 = property class="Bool (strict)"("Value"=TRUE) -> ()  [unwired: 2 in, 2 out]
                        }
                        frame 4 {
                          n296 = property class="Bool (strict)"("Value"=TRUE) -> ()  [unwired: 2 in, 2 out]
                        }
                        frame 5 {
                          n297 = property class="Bool (strict)"("Value"=TRUE) -> ()  [unwired: 2 in, 2 out]
                        }
                        frame 6 {
                          n298 = property class="Bool (strict)"("Value"=TRUE) -> ()  [unwired: 2 in, 2 out]
                        }
                        frame 7 {
                          n299 = property class="Bool (strict)"("Value"=TRUE) -> ()  [unwired: 2 in, 2 out]
                        }
                        frame 8 {
                          n300 = property class="Bool (strict)"("Value"=TRUE) -> ()  [unwired: 2 in, 2 out]
                        }
                        frame 9 {
                          n301 = property class="Bool (strict)"("Value"=TRUE) -> ()  [unwired: 2 in, 2 out]
                        }
                        frame 10 {
                          n302 = property class="Bool (strict)"("Value"=TRUE) -> ()  [unwired: 2 in, 2 out]
                        }
                      }
                    }
                  }
                  n303 = Subtract(x=w447, y=2) -> (x-y=w451:dbl)
                  n304 = Equal?(x=w453, y=w451) -> (x = y?=w450:bool)
                }
              }
            }
          }
          frame "Reset" {
            w474 = 1
            w481 = FALSE
            n305 = Bundle(w475, w476) -> (w480:cluster{i32[], i32[]})  [unwired: 1 in]
            n306 = property class="Bool (strict)"("Value"=w481) -> ()  [unwired: 2 in, 2 out]
            n307 = property class="Bool (strict)"("Value"=w481) -> ()  [unwired: 2 in, 2 out]
            n308 = property class="Bool (strict)"("Value"=w481) -> ()  [unwired: 2 in, 2 out]
            n309 = property on="Stay" class="Bool (strict)"("Value"=w481) -> ()  [unwired: 2 in, 2 out]
            n310 = property class="Bool (strict)"("Value"=w481) -> ()  [unwired: 2 in, 2 out]
            n311 = property class="Bool (strict)"("Value"=w481) -> ()  [unwired: 2 in, 2 out]
            n312 = property on="Switch" class="Bool (strict)"("Value"=w481) -> ()  [unwired: 2 in, 2 out]
            n313 = property class="Bool (strict)"("Value"=w481) -> ()  [unwired: 2 in, 2 out]
            n314 = property class="Bool (strict)"("Value"=w481) -> ()  [unwired: 2 in, 2 out]
            n315 = property class="Bool (strict)"("Value"=w481) -> ()  [unwired: 2 in, 2 out]
            n316 = property class="Bool (strict)"("Value"=w481) -> ()  [unwired: 2 in, 2 out]
            n317 = property class="Bool (strict)"("Value"=w481) -> ()  [unwired: 2 in, 2 out]
            n318 = Build Array(w480) -> (→"Manual Wins":cluster{i32[], i32[]}[])
            n319 = property on="Stay" class="Bool (strict)"("DisabledEnum"=w474) -> ()  [unwired: 2 in, 2 out]
            n320 = property on="Switch" class="Bool (strict)"("DisabledEnum"=w474) -> ()  [unwired: 2 in, 2 out]
          }
          frame "Switch" {
            w485 = 0
            w497 = 0
            n321 = event shown="[2] \"Stay\": Value Change" {
              selector: _ -> [_ _ _]
              dyn-events: _ -> [_ _ _]
              timeout: _ -> [_ _ _]
              tunnel: [_ w502 w506] -> w495
              tunnel: w499 -> [_ w501 w505]
              tunnel: w498 -> [_ w500 w504]
              event Timeout {
                n322 = event-data() -> ()  [unwired: 1 in, 3 out]
              }
              event "Switch": Value Change {
                n323 = event-data() -> ()  [unwired: 1 in, 4 out]
                n324 = Equal?(x=w500, y=w501) -> (x = y?=w503:bool)
                n325 = Not(x=w503) -> (.not. x?=w502:bool)
              }
              event "Stay": Value Change {
                n326 = event-data() -> ()  [unwired: 1 in, 4 out]
                n327 = Equal?(x=w504, y=w505) -> (x = y?=w506:bool)
              }
            }
            "Manual Win" <- w495
            n328 = property on="Stay" class="Bool (strict)"("DisabledEnum"=w485) -> ()  [unwired: 2 in, 2 out]
            n329 = property on="Switch" class="Bool (strict)"("DisabledEnum"=w485) -> ()  [unwired: 2 in, 2 out]
            n330 = Increment(x=w492) -> (x+1=w490:i32)
            n331 = Build Array (concatenate)(w491, w490) -> (w486:i32[])
            n332 = Boolean To (0,1)(Boolean=w495) -> (0, 1=w493:i16)
            n333 = Add(x=w494, y=w493) -> (x+y=w489:i32)
            n334 = Build Array (concatenate)(w488, w489) -> (w487:i32[])
          }
        }
      }
      n335 = property on="Manual Wins" class="XYGraph (strict)"("Visible"=w54) -> ()  [unwired: 2 in, 2 out]
      n336 = property class="Bool (strict)"("Visible"=w58, "DisabledEnum"=w65) -> ()  [unwired: 2 in, 2 out]
      n337 = property class="Bool (strict)"("Visible"=w59, "DisabledEnum"=w66) -> ()  [unwired: 2 in, 2 out]
      n338 = property class="Bool (strict)"("Visible"=w60, "DisabledEnum"=w67) -> ()  [unwired: 2 in, 2 out]
      n339 = property class="Bool (strict)"("Visible"=w61, "DisabledEnum"=w68) -> ()  [unwired: 2 in, 2 out]
      n340 = property class="Bool (strict)"("Visible"=w62, "DisabledEnum"=w69) -> ()  [unwired: 2 in, 2 out]
      n341 = property class="Bool (strict)"("Visible"=w64, "DisabledEnum"=w71) -> ()  [unwired: 2 in, 2 out]
      n342 = property class="Bool (strict)"("Visible"=w63, "DisabledEnum"=w70) -> ()  [unwired: 2 in, 2 out]
    }
  }
